vi "HatchCircle.vi"(10 "HatchPow":T6, 11 "CircHatch":T1={"Diameter"=1.0, "Angle"=45.0, "Offset"=0.1, "Spacing"=0.1} {"Spacing" format="%#_13g"; "Offset" format="%#_13g"; "Diameter" format="%#_13g"}) -> (3 "PathSupreme":T2)   [LabVIEW 2014]
uses:
  TypeDefs/PowerSpeed.ctl
  TypeDefs/PathSupreme.ctl
  PSup2SCAN/Sub/VelocityProfile.ctl
  PSup2SCAN/Sub/PathCut.ctl
  PSup2SCAN/Sub/Segment.ctl
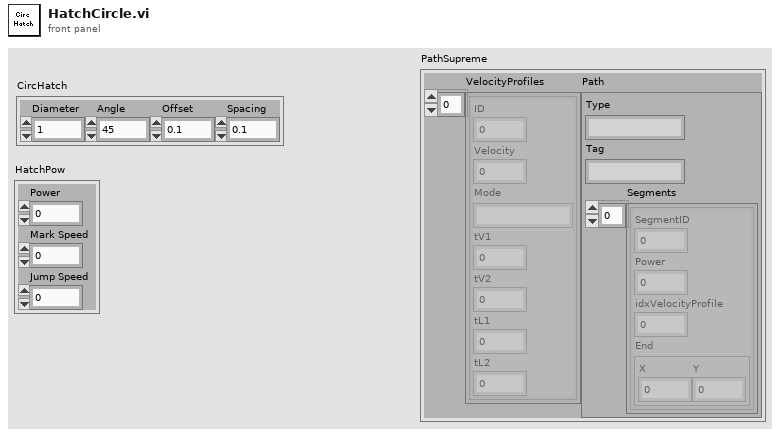
[diagram p1: front panel]
types:
  T1 = cluster{"Diameter":dbl, "Angle":sgl, "Offset":dbl, "Spacing":dbl}
  T2 = typedef "PathSupreme.ctl" = cluster{"VelocityProfiles":T3[], "Path":T4}
  T3 = typedef "VelocityProfile.ctl" = cluster{"ID":u32, "Velocity":dbl, "Mode":string, "tV1":u32, "tV2":u32, "tL1":u32, "tL2":u32}
  T4 = typedef "PathCut.ctl" = cluster{"Type":string, "Tag":string, "Segments":T5[]}
  T5 = typedef "Segment.ctl" = cluster{"SegmentID":u16, "Power":sgl, "idxVelocityProfile":u16, "End":cluster{"X":sgl, "Y":sgl}}
  T6 = typedef "PowerSpeed.ctl" = cluster{"Power":dbl, "Mark Speed":dbl, "Jump Speed":dbl}
  T7 = typedef "Point2DwSlope.ctl" = cluster{"X":sgl, "Y":sgl, "Slope":dbl}
  T8 = cluster{"Xmin":dbl, "Xmax":dbl, "Ymin":dbl, "Ymax":dbl}
  T9 = typedef "Poly2DwSlope.ctl" = cluster{"VertexArray":T7[]}
  T10 = cluster{"VertexArray":T7[], "OnOffAr":enum16{"On", "Off"}[]}
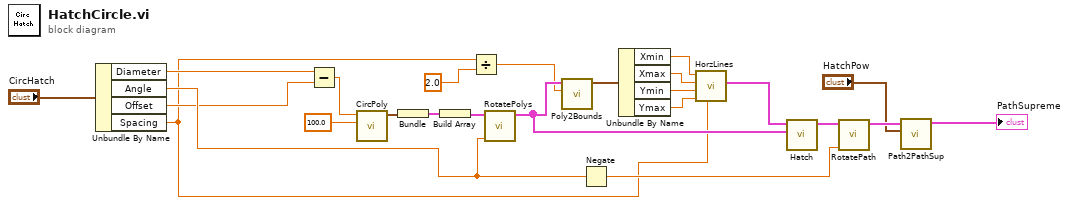
[diagram p0: block diagram]
diagram:
  n1 = Unbundle By Name("CircHatch") -> ("Diameter"=w9:dbl, "Angle"=w8:sgl, "Offset"=w7:dbl, "Spacing"=w5:dbl)
  n2 = Subtract(x=w9, y=w7) -> (x-y=w13:dbl)
  n3 = call "CircPoly.vi"("NumSides"=100.0, "Diameter"=w13) -> ("VertexArray"=w24:T7[])  [unwired: 9 in]
  n4 = Bundle("VertexArray"=w24) -> (w23:cluster{"VertexArray":T7[]})  [unwired: 1 in]
  n5 = Build Array(w23) -> (w17:cluster{"VertexArray":T7[]}[])
  n6 = Divide(x=w5, y=2.0) -> (x/y=w3:dbl)
  n7 = call "RotatePolys.vi"("Angle"=w8, "Polys"=w17) -> ("RotatedPolys"=w16:cluster{cluster{sgl, sgl, "Slope":dbl}[]}[])  [unwired: 9 in]
  n8 = call "Poly2Bounds.vi"("Border"=w3, "Polys"=w16) -> ("Bounds"=w6:T8)  [unwired: 9 in]
  n9 = Negate(x=w8) -> (-x=w14:sgl)
  n10 = Unbundle By Name(w6) -> ("Xmin"=w22:dbl, "Xmax"=w21:dbl, "Ymin"=w20:dbl, "Ymax"=w19:dbl)
  n11 = call "HorzLines.vi"("Spacing"=w5, "yMax"=w19, "yMin"=w20, "xMax"=w21, "xMin"=w22) -> ("Poly2D"=w18:T9)  [unwired: 5 in, 1 out]
  n12 = call "Hatch.vi"("Polys"=w16, "Hatch"=w18) -> ("Path"=w15:T10)  [unwired: 9 in]
  n13 = call "RotatePath.vi"("Angle"=w14, "Path"=w15) -> ("RotatedPath"=w12:T10)  [unwired: 9 in]
  n14 = call "Path2PathSup.vi"("PowerSpeed"="HatchPow", "Combined"=w12) -> ("PathSupreme"=→"PathSupreme":T2)  [unwired: 9 in]
